vi "Close_Instr.vi"(8 "error in (no error)":errorcluster caption="entrée d'erreur (pas d'erreur)", 11 "Class Instrument Printer en entrée":refnum<class "Class Instrument Printer.lvclass">) -> (0 "error out":errorcluster caption="sortie d'erreur", 3 "Class Instrument Printer en sortie":refnum<class "Class Instrument Printer.lvclass">)   [LabVIEW 2020, in "Library Instrument & Equipement.lvlib" / "Library Instruments.lvlib" / "Class Instrument Printer.lvclass"]
doc: "releases and closes an instrument"
uses:
  Class Instrument Printer.lvclass
  Class Instrument Printer.lvclass/Class Instrument Printer.ctl
  Instrument (Default)/Class Instrument (Default).lvclass
  Printer/Printer (Default)/Class Printer (Default).lvclass
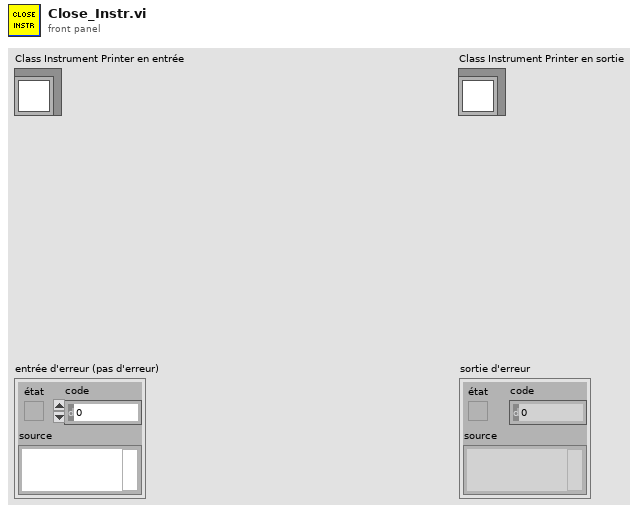
[diagram p1: front panel]
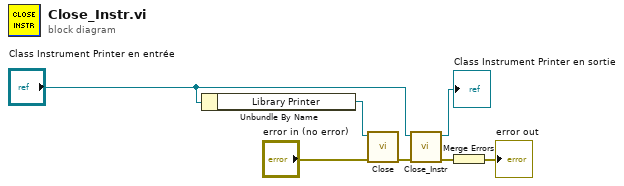
[diagram p0: block diagram]
diagram:
  n1 = Unbundle By Name("Class Instrument Printer en entrée") -> ("Library Printer"=w5:refnum<class "Class Printer (Default).lvclass">)
  n2 = call-dynamic "Close.vi"("error in (no error)"="error in (no error)", "Class Printer (Default) en entrée"=w5) -> ("error out"=w6:errorcluster)  [unwired: 8 in, 1 out]
  n3 = call-parent "Close_Instr.vi"("error in (no error)"=w6, "Class Instrument (Default) en entrée"="Class Instrument Printer en entrée") -> ("error out"=w1:errorcluster, "Class Instrument (Default) en sortie"=→"Class Instrument Printer en sortie":refnum<class "Class Instrument Printer.lvclass">)  [unwired: 8 in]
  n4 = Merge Errors(w1) -> (→"error out":errorcluster)
